vi "Check.vi"(8 "error in (no error)":errorcluster, 10 "Encoded string":string, 11 "Encoding in":refnum<class "CConfig UCS-16 Encoding.lvclass">) -> (0 "error out":errorcluster, 1 "Match?":bool, 2 "Encoded string":string, 3 "Encoding out":refnum<class "CConfig UCS-16 Encoding.lvclass">)   [LabVIEW 2013, in "CConfig UCS-16 Encoding.lvclass"]
doc: "Copyright 2018, Carya Automatisering, Wiebe Walstra."
uses:
  CConfig UCS-16 Encoding.lvclass
  CConfig UCS-16 Encoding.lvclass/CConfig UCS-16 Encoding.ctl
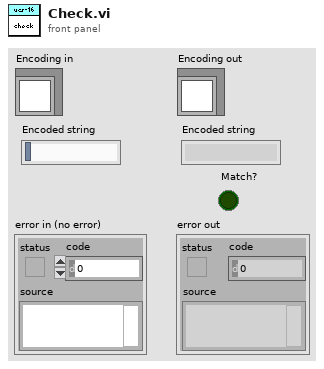
[diagram p1: front panel]
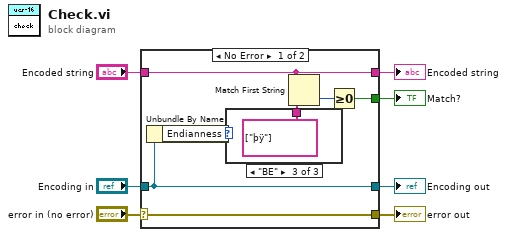
[diagram p0: block diagram]
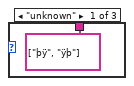
[diagram p2: hidden frame]
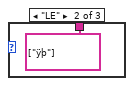
[diagram p3: hidden frame]
diagram:
  n1 = case shown="No Error" "error in (no error)" {
    selector: "error in (no error)" -> [w14 w19]
    tunnel: [w14 w19] -> w6
    tunnel: "Encoded string" -> [w12 w20]
    tunnel: [w12 w20] -> w4
    tunnel: [w10 _] -> w3
    tunnel: [w9 w18] -> w2
    tunnel: "Encoding in" -> [w9 w18]
    frame No Error {
      n2 = Unbundle By Name(w9) -> ("Endianness"=w8:enum16{"BE", "LE", "unknown"})
      n3 = case shown="\"BE\"" w8 {
        tunnel: [string[] ["þÿ", "ÿþ"] string[] ["ÿþ"] string[] ["þÿ"]] -> w11
        frame "unknown" {
        }
        frame "LE" {
        }
        frame "BE" {
        }
      }
      n4 = Match First String(2:w11, 3:w12) -> (0:w13:i32)  [unwired: 1 out]
      n5 = Greater Or Equal To 0?(x=w13) -> (x >= 0?=w10:bool)
    }
    frame Error {
    }
  }
  "error out" <- w6
  "Encoding out" <- w2
  "Encoded string" <- w4
  "Match?" <- w3
